vi "get.vi"(1 "Numeric 2":i32) -> (0 "SHOW":dbl[][](array[numeric]))   [LabVIEW 2014]
panel:
  out "Array":dbl[][](array[numeric])
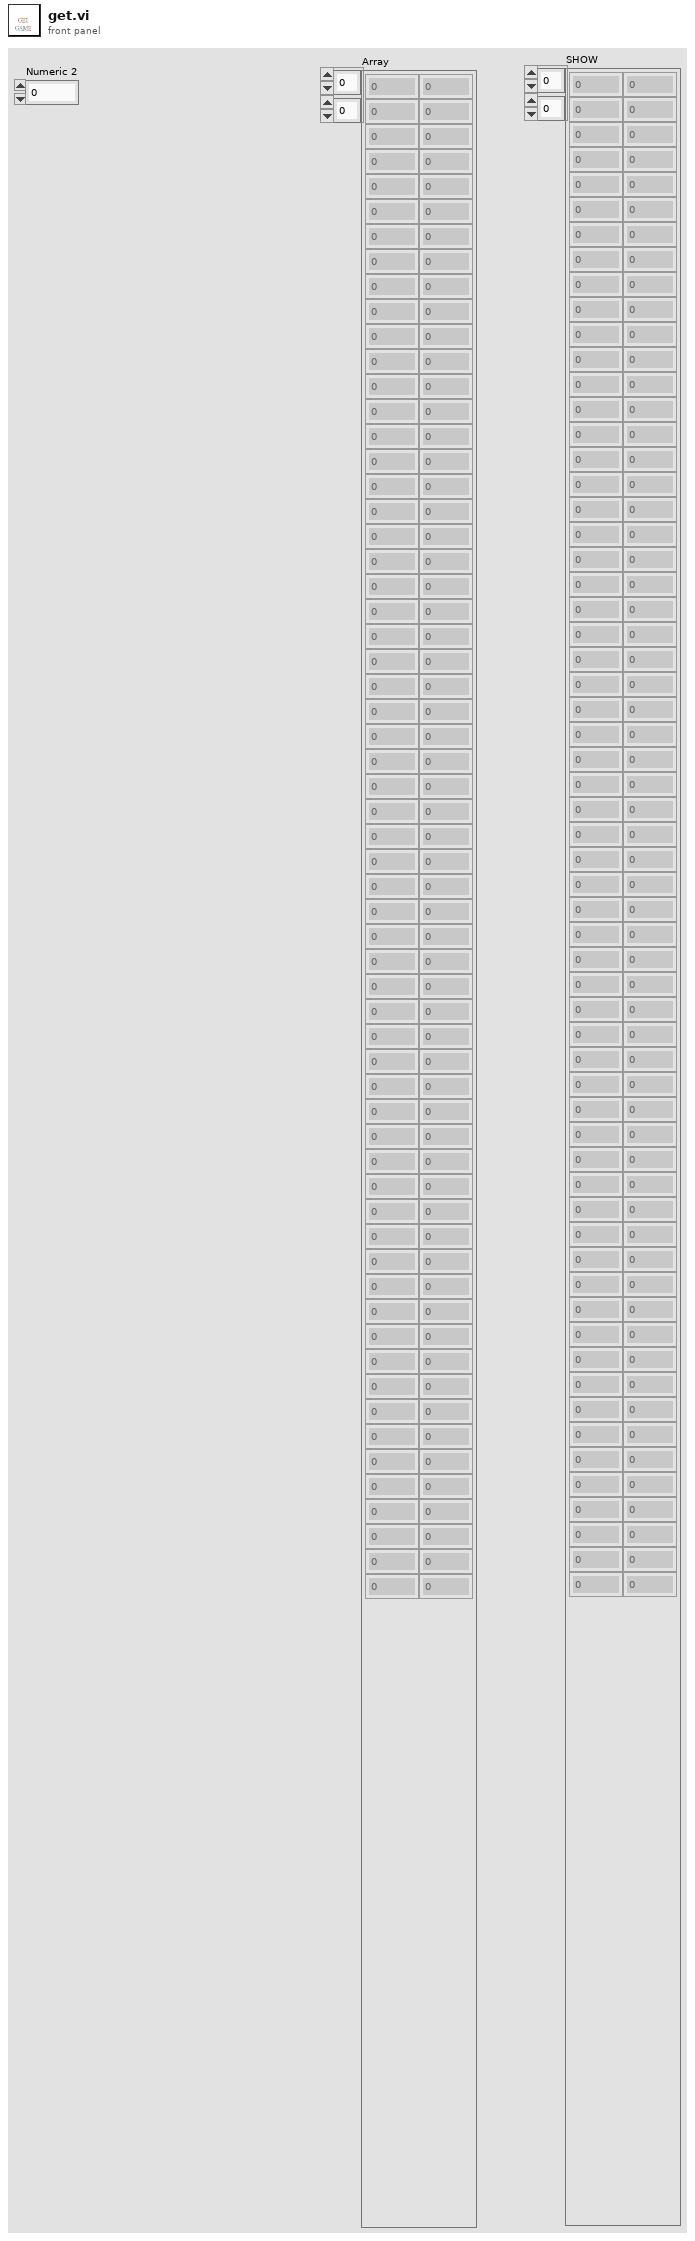
[diagram p1: front panel]
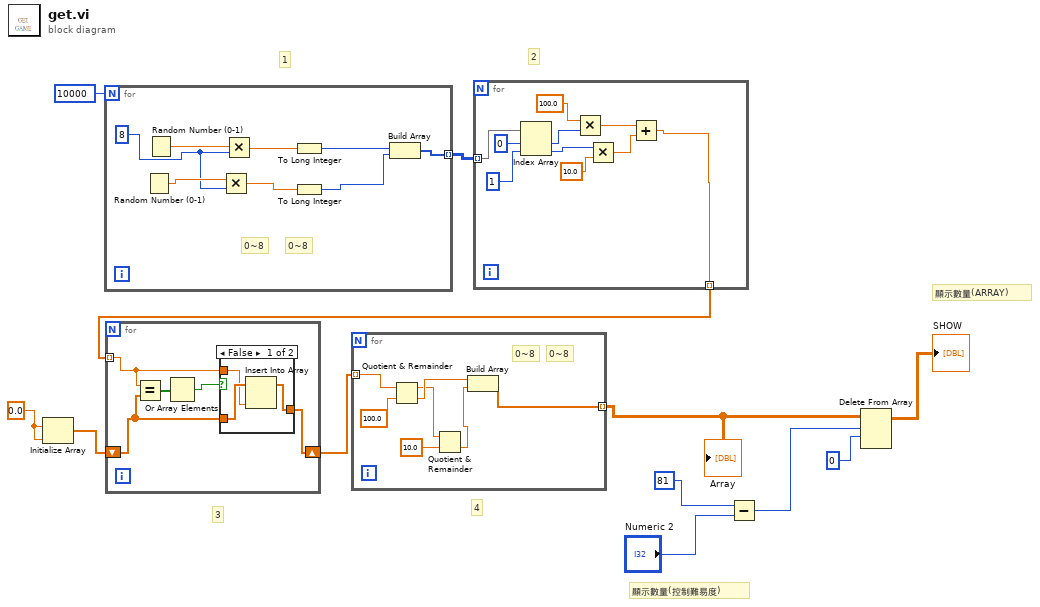
[diagram p0: block diagram]
diagram:
  w10 = 0.0 ("element")
  # "顯示數量(ARRAY)"
  # "顯示數量(控制難易度)"
  # "3"
  # "4"
  # "2"
  # "1"
  n1 = Initialize Array(w10, w10) -> (w9:dbl[])
  n2 = for {
    N: 10000 -> [_]
    tunnel: [w18] -> w11 mode=indexing
    w17 = 8
    # "0~8"
    # "0~8"
    n3 = Random Number (0-1)() -> (number: 0 to 1=w20:dbl)
    n4 = Random Number (0-1)() -> (number: 0 to 1=w19:dbl)
    n5 = Multiply(x=w20, y=w17) -> (x*y=w15:dbl)
    n6 = Multiply(x=w19, y=w17) -> (x*y=w14:dbl)
    n7 = To Long Integer(number=w14) -> (32bit integer=w13:i32)
    n8 = To Long Integer(number=w15) -> (32bit integer=w16:i32)
    n9 = Build Array(w13, w16) -> (w18:i32[])
  }
  n10 = for {
    tunnel: w11 -> [w30] mode=indexing
    tunnel: [w21] -> w7 mode=indexing
    n11 = Index Array(array=w30, index #1=0 ("index"), index #2=1 ("index")) -> (element #1=w27:i32, element #2=w25:i32)
    n12 = Multiply(x=100.0, y=w27) -> (x*y=w23:dbl)
    n13 = Multiply(x=w25, y=10.0) -> (x*y=w22:dbl)
    n14 = Add(x=w23, y=w22) -> (x+y=w21:dbl)
  }
  n15 = for {
    shift-right: [w31] -> w8
    shift-left: w9 -> [w32]
    tunnel: w7 -> [w34] mode=indexing
    n16 = Equal?(x=w34, y=w32) -> (x = y?=w35:bool[])
    n17 = Or Array Elements(Boolean array=w35) -> (logical OR=w33:bool)
    n18 = case shown="False" w33 {
      tunnel: w34 -> [w37 _]
      tunnel: w32 -> [w38 w39]
      tunnel: [w36 w39] -> w31
      frame False {
        n19 = Insert Into Array(array=w38, new element=w37) -> (w36:dbl[])  [unwired: 1 in]
      }
      frame True {
      }
    }
  }
  n20 = for {
    tunnel: w8 -> [w46] mode=indexing
    tunnel: [w44] -> w4 mode=indexing
    # "0~8"
    # "0~8"
    n21 = Quotient & Remainder(x=w46, y=100.0) -> (x-y*floor(x/y)=w41:dbl, floor(x/y)=w43:dbl)
    n22 = Quotient & Remainder(x=w41, y=10.0) -> (floor(x/y)=w40:dbl)  [unwired: 1 out]
    n23 = Build Array(w43, w40) -> (w44:dbl[])
  }
  "Array" <- w4
  n24 = Subtract(x=81, y="Numeric 2") -> (x-y=w2:i32)
  n25 = Delete From Array(array=w4, length=w2, index (row)=0) -> (array with subset deleted=→"SHOW":dbl[][])  [unwired: 1 in, 1 out]
